vi "test Open Enqueue Close.vi"(8 "error in (no error)":errorcluster, 11 "TestCase in":refnum<class "Message Queue Test Case.lvclass">) -> (0 "error out":errorcluster, 3 "TestCase out":refnum<class "Message Queue Test Case.lvclass">)   [LabVIEW 2017, in "Message Queue Test Case.lvclass"]
uses:
  Message Queue Test Case.lvclass
  Support/Messages/Test Message/Test Message.lvclass
  C:/github/niveristand-custom-device-message-library/Source/Message/Abstract Message/Abstract Message.lvclass
  Message Queue Test Case.lvclass/Message Queue Test Case.ctl
  Message Queue/Abstract Message Queue/Abstract Message Queue.lvclass
  <vilib>/addons/_JKI Toolkits/VI Tester/TestCase.llb/TestCase.lvclass
  C:/Program Files (x86)/National Instruments/LabVIEW 2017/vi.lib/addons/_JKI Toolkits/VI Tester/TestCase.llb/TestCase.lvclass
panel:
  out "Data":string
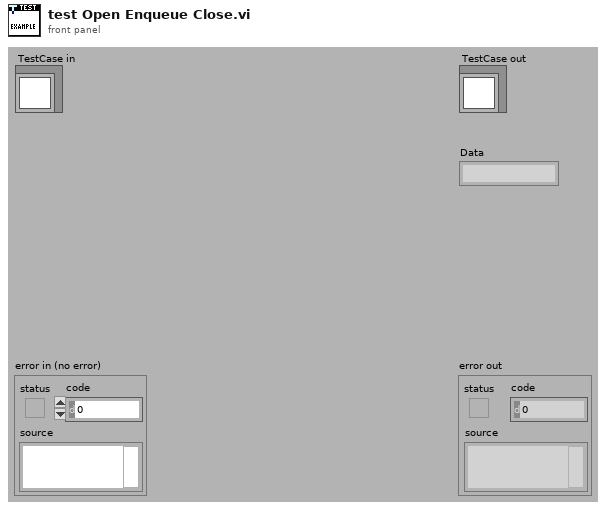
[diagram p1: front panel]
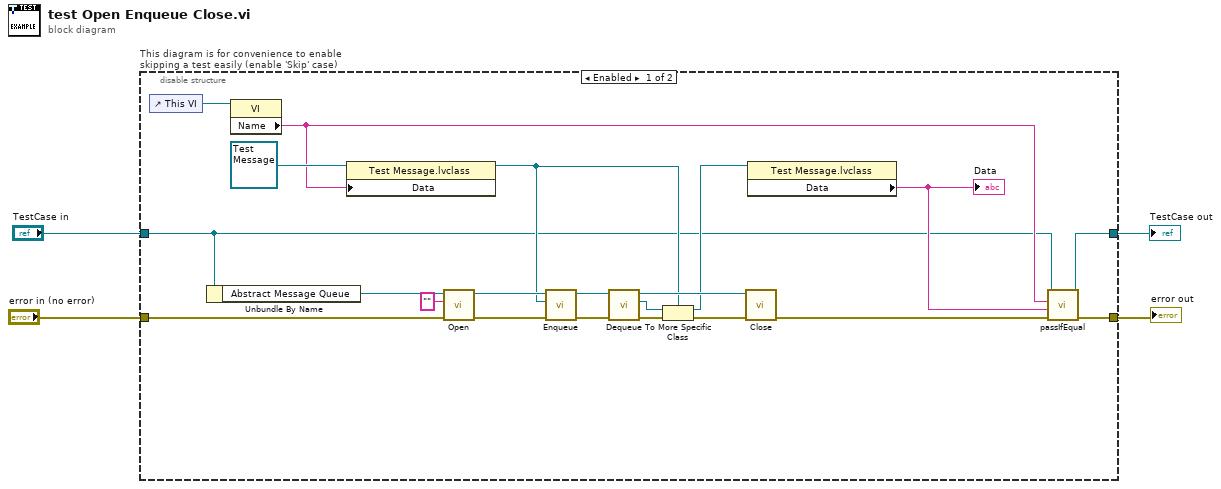
[diagram p0: block diagram]
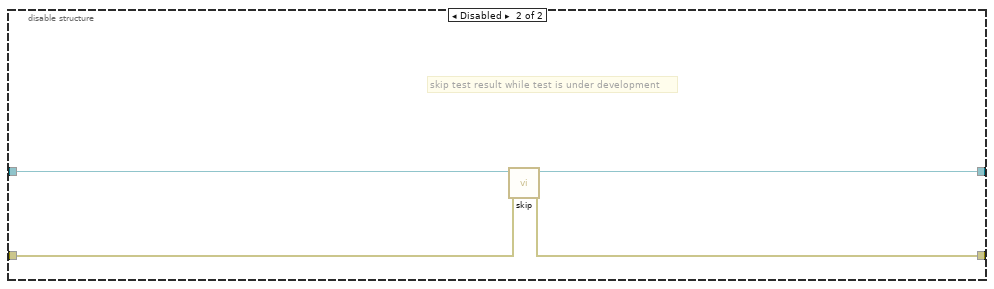
[diagram p2: hidden frame]
diagram:
  n1 = disable-structure "This diagram is for convenience to enable skipping a test easily (enable 'Skip' case)" shown="Enabled" {
    disable-tunnel: "TestCase in" -> [w10 w29]
    disable-tunnel: [w9 w27] -> w1
    disable-tunnel: [w8 w28] -> w3
    disable-tunnel: "error in (no error)" -> [w25 w26]
    frame Enabled {
      n2 = control-ref of="This VI"() -> (w17:refnum<vi>)
      n3 = Unbundle By Name(w10) -> ("Abstract Message Queue"=w24:refnum<class "Abstract Message Queue.lvclass">)
      n4 = property class="VI"(reference=w17) -> ("Name"=w12:string)  [unwired: 1 in, 2 out]
      n5 = property class="Test Message.lvclass"(reference=refnum<class "Test Message.lvclass"> refnum ("Test Message.lvclass"), "Data"=w12) -> (reference out=w15:refnum<class "Test Message.lvclass">)  [unwired: 1 in, 1 out]
      n6 = call-dynamic "Open.vi"("error in (no error)"=w25, "name (unnamed)"="", "Abstract Message Queue in"=w24) -> ("error out"=w23:errorcluster, "Abstract Message Queue out"=w22:refnum<class "Abstract Message Queue.lvclass">)  [unwired: 7 in]
      n7 = call-dynamic "Enqueue.vi"("error in (no error)"=w23, "Message in"=w15, "Abstract Message Queue in"=w22) -> ("error out"=w21:errorcluster, "Abstract Message Queue out"=w20:refnum<class "Abstract Message Queue.lvclass">)  [unwired: 7 in]
      n8 = call-dynamic "Dequeue.vi"("error in (no error)"=w21, "Abstract Message Queue in"=w20) -> ("error out"=w6:errorcluster, "Message out"=w16:refnum<class "Abstract Message.lvclass">, "Abstract Message Queue out"=w19:refnum<class "Abstract Message Queue.lvclass">)  [unwired: 7 in]
      n9 = To More Specific Class(target class=w15, reference=w16, error in=w6) -> (specific class reference=w14:refnum<class "Test Message.lvclass">, error out=w5:errorcluster)
      n10 = call-dynamic "Close.vi"("error in (no error)"=w5, "Abstract Message Queue in"=w19) -> ("error out"=w13:errorcluster)  [unwired: 8 in, 1 out]
      n11 = property class="Test Message.lvclass"(reference=w14) -> ("Data"=w11:string)  [unwired: 1 in, 2 out]
      "Data" <- w11
      n12 = call-dynamic "passIfEqual.vi"("error in (no error)"=w13, "y"=w11, "x"=w12, "TestCase in"=w10) -> ("error out"=w8:errorcluster, "TestCase out"=w9:refnum<class "Message Queue Test Case.lvclass">)  [unwired: 6 in]
    }
    frame Disabled {
      # "skip test result while test is under development"
      n13 = call <vilib>:"skip.vi"("error in (no error)"=w26, "TestCase in"=w29) -> ("error out"=w28:errorcluster, "TestCase out"=w27:refnum<class "Message Queue Test Case.lvclass">)  [unwired: 8 in]
    }
  }
  "error out" <- w3
  "TestCase out" <- w1
